vi "Mouse UP.vi"(8 "error in (no error)":errorcluster, 10 "Cell Position":T1, 11 "MouseHandle in":refnum<class "MouseHandle.lvclass">) -> (0 "error out":errorcluster, 3 "MouseHandle out":refnum<class "MouseHandle.lvclass">)   [LabVIEW 2021, in "MouseHandle.lvlib" / "MouseHandle.lvclass"]
uses:
  <userlib>/John_Lib/Interfaces/MouseHandle/MouseHandle.lvclass
  <vilib>/Utility/miscctls.llb/LVRowAndColumnTypeDef.ctl
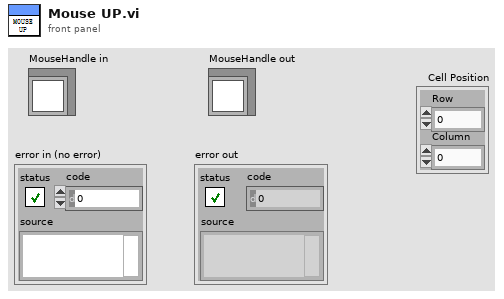
[diagram p1: front panel]
types:
  T1 = typedef "LVRowAndColumnTypeDef.ctl" = cluster{"Row":i32, "Column":i32}
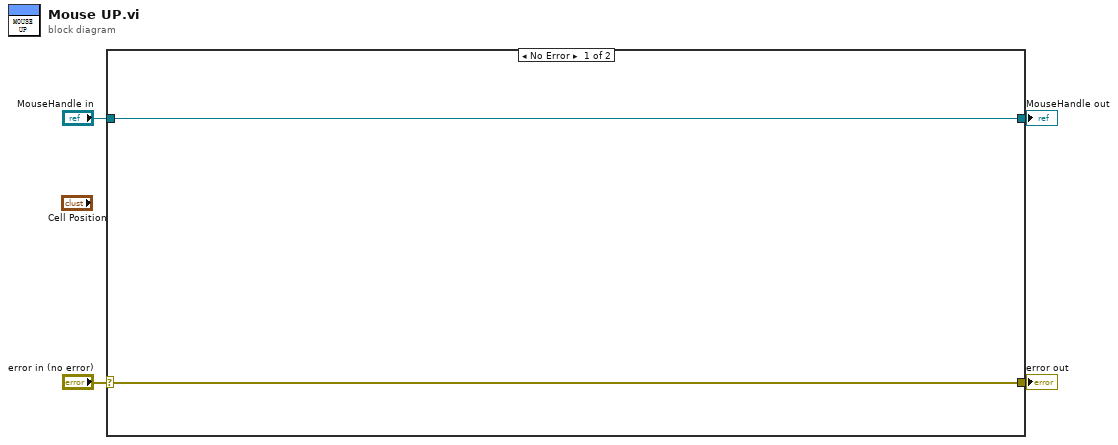
[diagram p0: block diagram]
diagram:
  n1 = case shown="No Error" "error in (no error)" {
    selector: "error in (no error)" -> [w5 w8]
    tunnel: [w5 w8] -> w3
    tunnel: [w6 w7] -> w1
    tunnel: "MouseHandle in" -> [w6 w7]
    frame No Error {
    }
    frame Error {
    }
  }
  "error out" <- w3
  "MouseHandle out" <- w1
